vi "Introspection Input.vi"(8 "error in (no error)":errorcluster, 11 "session id in":i32) -> (0 "error out":errorcluster, 2 "Introspection Input":T1, 3 "session id out":i32)   [LabVIEW 2017, in "libonnx_wrapper.lvlib"]
uses:
  libonnx_wrapper.lvlib
  TypeDef/Introspection.ctl
  TypeDef/IO.ctl
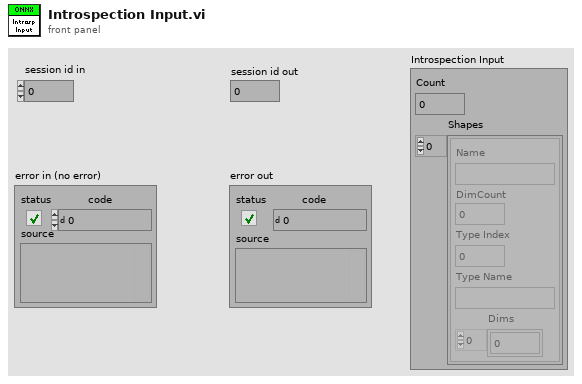
[diagram p1: front panel]
types:
  T1 = typedef "libonnx_wrapper.lvlib/Introspection.ctl" = cluster{"Count":i32, "Shapes":T2[]}
  T2 = typedef "libonnx_wrapper.lvlib/IO.ctl" = cluster{"Name":string, "DimCount":i32, "Type Index":i32, "Type Name":string, "Dims":i64[]}
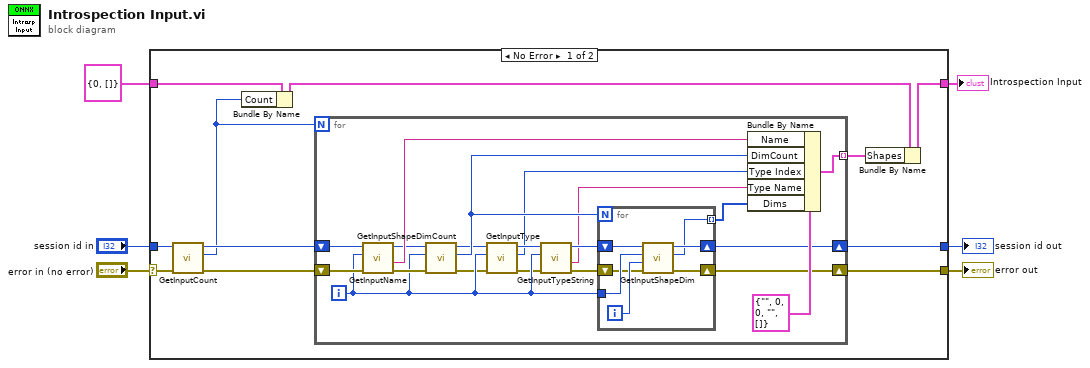
[diagram p0: block diagram]
diagram:
  n1 = case shown="No Error" "error in (no error)" {
    selector: "error in (no error)" -> [w16 w46]
    tunnel: "session id in" -> [w17 w47]
    tunnel: [w14 w47] -> w4
    tunnel: [w12 w46] -> w3
    tunnel: [w8 w45] -> w1
    tunnel: T1 {"Count"=0, "Shapes"=[]} ("Introspection") -> [w10 w45]
    frame No Error {
      n2 = call "GetInputCount.vi"("error in (no error)"=w16, "session id in"=w17) -> ("error out"=w13:errorcluster, "InputCount"=w11:i32, "session id out"=w15:i32)  [unwired: 7 in]
      n3 = Bundle By Name(cluster=w10, "Count"=w11) -> (w9:T1)
      n4 = for {
        N: w11 -> [_]
        shift-right: [w21] -> w14
        shift-left: w15 -> [w37]
        shift-right: [w22] -> w12
        shift-left: w13 -> [w36]
        tunnel: [w33] -> w7 mode=indexing
        i -> [w29]
        n5 = call "GetInputName.vi"("error in (no error)"=w36, "index"=w29, "session id in"=w37) -> ("error out"=w31:errorcluster, "InputName"=w35:string, "session id out"=w32:i32)  [unwired: 5 in, 1 out]
        n6 = call "GetInputShapeDimCount.vi"("error in (no error)"=w31, "inputIndex"=w29, "session id in"=w32) -> ("error out"=w26:errorcluster, "InputShapeDimCount"=w30:i32, "session id out"=w28:i32)  [unwired: 6 in]
        n7 = call "GetInputType.vi"("error in (no error)"=w26, "inputIndex"=w29, "session id in"=w28) -> ("error out"=w25:errorcluster, "InputTypeIndex"=w19:i32, "session id out"=w27:i32)  [unwired: 6 in]
        n8 = call "GetInputTypeString.vi"("error in (no error)"=w25, "index"=w29, "session id in"=w27) -> ("error out"=w23:errorcluster, "InputTypeName"=w18:string, "session id out"=w24:i32)  [unwired: 5 in, 1 out]
        n9 = for {
          N: w30 -> [_]
          shift-right: [w40] -> w21
          shift-left: w24 -> [w41]
          shift-right: [w42] -> w22
          shift-left: w23 -> [w38]
          tunnel: w29 -> [w43]
          tunnel: [w39] -> w20 mode=indexing
          i -> [w44]
          n10 = call "GetInputShapeDim.vi"("error in (no error)"=w38, "dimIndex"=w44, "inputIndex"=w43, "session id in"=w41) -> ("error out"=w42:errorcluster, "InputShapeDim"=w39:i64, "session id out"=w40:i32)  [unwired: 5 in]
        }
        n11 = Bundle By Name(cluster=T2 {"Name"="", "DimCount"=0, "Type Index"=0, "Type Name"="", "Dims"=[]} ("Shape"), "Name"=w35, "DimCount"=w30, "Type Index"=w19, "Type Name"=w18, "Dims"=w20) -> (w33:T2)
      }
      n12 = Bundle By Name(cluster=w9, "Shapes"=w7) -> (w8:T1)
    }
    frame Error {
    }
  }
  "error out" <- w3
  "session id out" <- w4
  "Introspection Input" <- w1
